vi "HT3_Create.vi"(4 "Image Header in":T3, 5 "Save pt3":bool=TRUE, 6 "Measurement Type":T2(ring)=enum."Point Measurement", 7 "overwrite existing":bool, 8 "error in":errorcluster, 9 "Comment":string, 10 "ht3 Header in":T4={"Comment"="", "Binning"=0, "Offset"=0, "AcquisitionTime (ms)"=0, "HardwareSerial"=0, "SyncDivider"=0, "Resolution (ps)"=0.0, "InpRate0"=0, "InpRate1"=0, "CFD Settings"={"Sync Level"=150, "Sync ZeroX"=10, "Sync Offset"=-1000, "Chan Settings"=[{"CHx Level"=50, "CHx ZeroX"=10, "CHx Offset"=0}, {"CHx Level"=50, "CHx ZeroX"=10, "CHx Offset"=0}, {"CHx Level"=50, "CHx ZeroX"=10, "CHx Offset"=0}, {"CHx Level"=50, "CHx ZeroX"=10, "CHx Offset"=0}]}, "ModuleInfo"=[], "BaseResolution (ps)"=0.0, "RefClockSource"=0, "ChanInfo"=[], "SyncRate"=0, "InputsEnabled"=0}, 11 "File Path":path) -> (0 "error out":errorcluster, 2 "FileHeaderPos":T1, 3 "refnum out":refnum<file>)   [LabVIEW 2013]
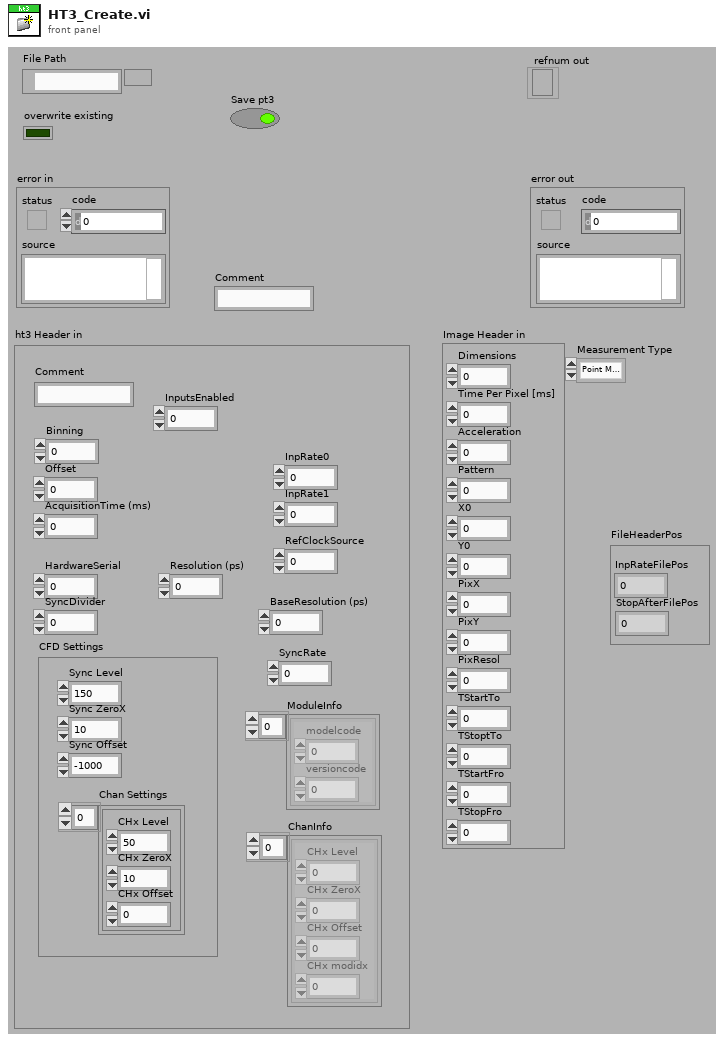
[diagram p1: front panel]
types:
  T1 = cluster{"InpRateFilePos":i64, "StopAfterFilePos":i64}
  T2 = enum16{"not a pt3 File", "Image File", "Point Measurement", "Auto Point", "Line Scan"}
  T3 = cluster{"Dimensions":i32, "Time Per Pixel [ms]":dbl, "Acceleration":i32, "Pattern":i32, "X0":sgl, "Y0":sgl, "PixX":i32, "PixY":i32, "PixResol":sgl, "TStartTo":sgl, "TStoptTo":sgl, "TStartFro":sgl, "TStopFro":sgl}
  T4 = cluster{"Comment":string, "Binning":i32, "Offset":i32, "AcquisitionTime (ms)":i32, "HardwareSerial":i32, "SyncDivider":i32, "Resolution (ps)":dbl, "InpRate0":i32, "InpRate1":i32, "CFD Settings":cluster{"Sync Level":i32, "Sync ZeroX":i32, "Sync Offset":i32, "Chan Settings":cluster{"CHx Level":i32, "CHx ZeroX":i32, "CHx Offset":i32}[]}, "ModuleInfo":cluster{"modelcode":i32, "versioncode":i32}[], "BaseResolution (ps)":dbl, "RefClockSource":i32, "ChanInfo":cluster{"CHx Level":i32, "CHx ZeroX":i32, "CHx Offset":i32, "CHx modidx":i32}[], "SyncRate":i32, "InputsEnabled":i64}
  T5 = enum16{"big-endian, network order", "native, host order", "little-endian"}
  T6 = enum16{"open", "replace", "create", "open or create", "replace or create", "replace or create with confirmation"}
  T7 = cluster{"NumberOfCurves":i32, "Bits per Record":i32, "ActiveCurve":i32, "MeasurementMode (3 = T3)":i32, "f":i32, "Binning":i32, "Resolution (ps)":dbl, "Offset":i32, "AcquisitionTime (ms)":i32, "StopAt":u32, "StopOnOvfl":i32, "Restart":i32, "DisplayLinLog":i32, "DisplayTimeAxisFrom":i32, "DisplayTimeAxisTo":i32, "DisplayCountAxisFrom":i32, "DisplayCountAxisTo":i32}
  T8 = cluster{"Sync Level":i32, "Sync ZeroX":i32, "Sync Offset":i32, "Chan Settings":cluster{"CHx Level":i32, "CHx ZeroX":i32, "CHx Offset":i32}[]}
  T9 = cluster{"CHx Level":i32, "CHx ZeroX":i32, "CHx Offset":i32, "CHx modidx":i32}[]
  T10 = cluster{"BaseResolution (ps)":dbl, "InputsEnabled":i64, i32, "RefClockSource":i32, "ExtDevices":i32, "MarkerSettings":i32, "SyncDivider":i32, "Sync Level":i32, "Sync ZeroX":i32, "Sync Offset":i32}
  T11 = cluster{"SyncRate":i32, "StopAfter":i32, "StopReason":i32, "f":i32, "NumRecords":i64}
  T12 = cluster{"offset (in bytes)":i64, "offset (in bytes)":i64}
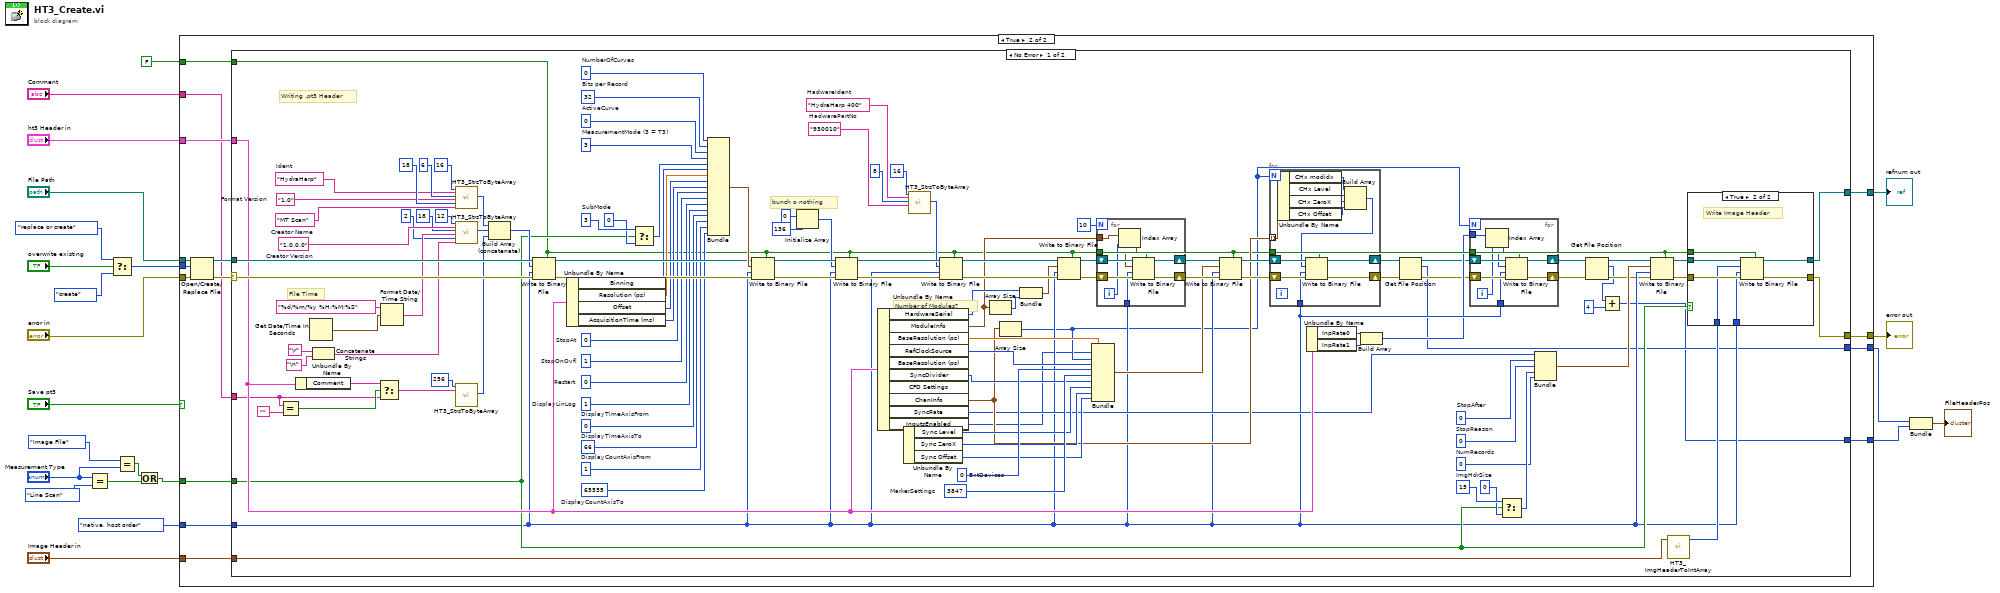
[diagram p0: block diagram]
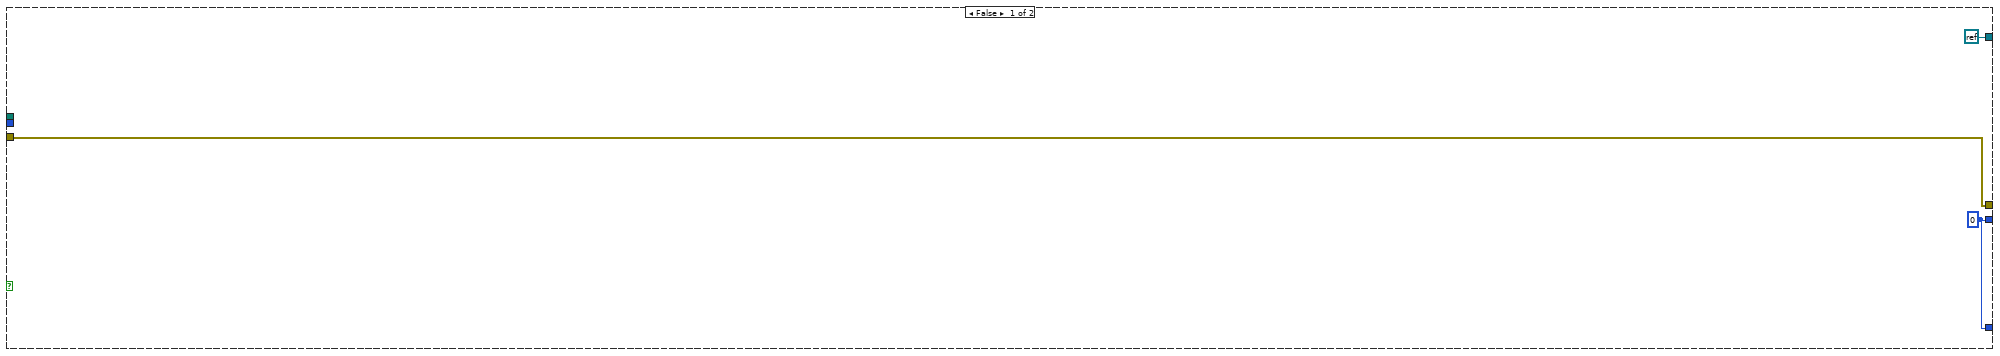
[diagram p2: hidden frame]
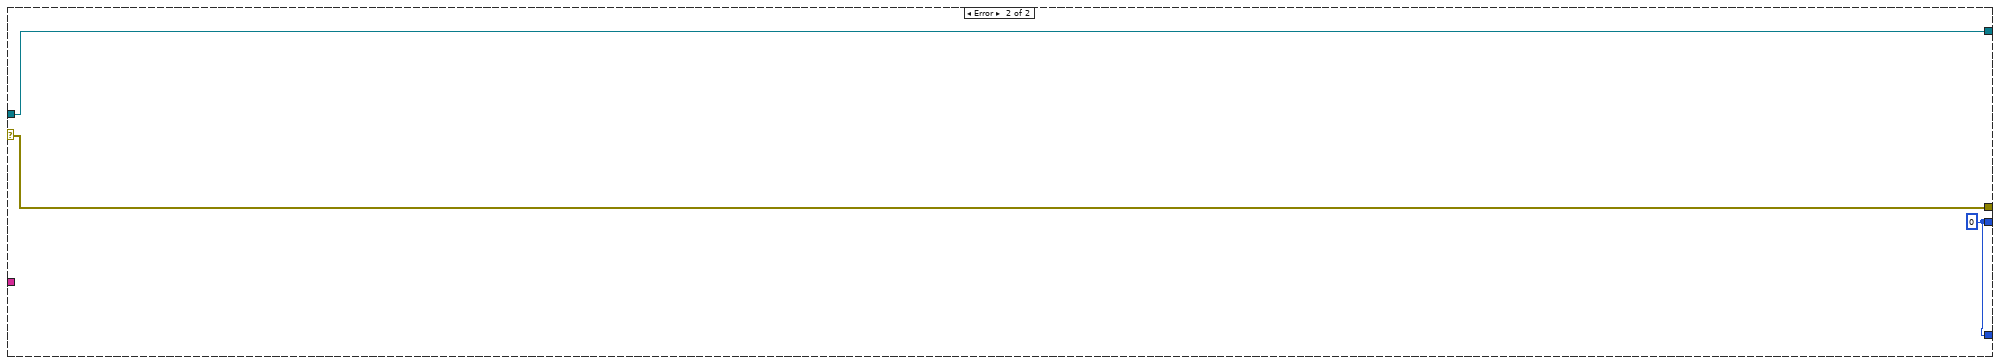
[diagram p4: hidden frame]
diagram:
  n1 = Equal?(x="Measurement Type", y=T2."Line Scan") -> (x = y?=w3:bool)
  n2 = Select(t=T6."replace or create" ("operation (0:open)"), s="overwrite existing", f=T6."create" ("operation (0:open)")) -> (s? t:f=w19:T6)
  n3 = Equal?(x=T2."Image File" ("y"), y="Measurement Type") -> (x = y?=w2:bool)
  n4 = Or(x=w2, y=w3) -> (x .or. y?=w1:bool)
  n5 = case shown="True" "Save pt3" {
    tunnel: "File Path" -> [_ w41]
    tunnel: w19 -> [_ w40]
    tunnel: "error in" -> [w26 w39]
    tunnel: [w26 w37] -> w17
    tunnel: [refnum<k0> refnum w35] -> w16
    tunnel: "ht3 Header in" -> [_ w34]
    tunnel: T5."native, host order" ("byte order (0:big-endian, network order)") -> [_ w33]
    tunnel: FALSE ("prepend array or string size? (T)") -> [_ w32]
    tunnel: "Comment" -> [_ w31]
    tunnel: w1 -> [_ w30]
    tunnel: "Image Header in" -> [_ w29]
    tunnel: [w24 w28] -> w9
    tunnel: [w24 w27] -> w8
    frame False {
      w24 = i64 0 ("offset (in bytes)")
    }
    frame True {
      n6 = Open/Create/Replace File(file path (use dialog)=w41, error in=w39, operation (0:open)=w40) -> (refnum out=w36:refnum<file>, error out=w38:errorcluster)  [unwired: 4 out]
      n7 = case shown="No Error" w38 {
        selector: w38 -> [w162 w204]
        tunnel: [w91 w204] -> w37
        tunnel: w36 -> [w161 w203]
        tunnel: [w89 w203] -> w35
        tunnel: w34 -> [w107 _]
        tunnel: w33 -> [w58 _]
        tunnel: w32 -> [w59 _]
        tunnel: w31 -> [w100 _]
        tunnel: w30 -> [w93 _]
        tunnel: w29 -> [w94 _]
        tunnel: [w44 w202] -> w28
        tunnel: [w43 w202] -> w27
        frame No Error {
          w74 = 3847  # MarkerSettings
          w75 = 0  # ExtDevices
          w96 = 15  # ImgHdrSize
          w60 = i64 0  # NumRecords
          w105 = 0  # StopReason
          w106 = 0  # StopAfter
          w113 = "930010"  # HadwarePartNo
          w115 = "HydraHarp 400"  # HadwareIdent
          w124 = 65535  # DisplayCountAxisTo
          w125 = 1  # DisplayCountAxisFrom
          w126 = 66  # DisplayTimeAxisTo
          w127 = 0  # DisplayTimeAxisFrom
          w128 = 1  # DisplayLinLog
          w129 = 0  # Restart
          w130 = 1  # StopOnOvfl
          w131 = u32 0  # StopAt
          w98 = 3  # SubMode
          w135 = 3  # MeasurementMode (3 = T3)
          w136 = 0  # ActiveCurve
          w86 = 32  # Bits per Record
          w87 = 0  # NumberOfCurves
          w150 = "1.0.0.0"  # Creator Version
          w151 = "MT Scan"  # Creator Name
          w152 = "1.0"  # Format Version
          w153 = "HydraHarp"  # Ident
          # "Number of Modules?"
          # "bunch o nothing"
          # "File Time"
          # "Writing .pt3 Header"
          n8 = Equal?(x=w100, y="") -> (x = y?=w102:bool)
          n9 = Unbundle By Name(w107) -> ("Comment"=w101:string)
          n10 = Get Date/Time In Seconds() -> (seconds since 1Jan1904=w158:timestamp)
          n11 = Concatenate Strings("\r", "\n") -> (w148:string)
          n12 = Select(t=w101, s=w102, f=w100) -> (s? t:f=w99:string)
          n13 = Format Date/Time String(time format string (%c)="%d/%m/%y %H:%M:%S", seconds (now)=w158) -> (date/time string=w149:string)  [unwired: 1 out]
          n14 = call "HT3_StrsToByteArray.vi"("Length"=16, "String"=w153, "Length 2"=6 ("Length"), "String 2"=w152, "Length 3"=18 ("Length"), "String 3"=w151) -> ("Byte Array"=w144:u8[])  [unwired: 1 in, 12 out]
          n15 = call "HT3_StrsToByteArray.vi"("Length"=12, "String"=w150, "Length 2"=18 ("Length"), "String 2"=w149, "Length 3"=2 ("Length"), "String 3"=w148) -> ("Byte Array"=w143:u8[])  [unwired: 1 in, 12 out]
          n16 = call "HT3_StrsToByteArray.vi"("Length"=256, "String"=w99) -> ("Byte Array"=w141:u8[])  [unwired: 5 in, 12 out]
          n17 = Build Array (concatenate)(w144, w143, w141) -> (w140:u8[])
          n18 = Write to Binary File(file (use dialog)=w161, data=w140, error in=w162, 5:w59, 9:w58) -> (refnum out=w137:refnum<file>, error out=w138:errorcluster)  [unwired: 2 out]
          n19 = Unbundle By Name(w107) -> ("Binning"=w84:i32, "Resolution (ps)"=w134:dbl, "Offset"=w133:i32, "AcquisitionTime (ms)"=w132:i32)
          n20 = Select(t=w98, s=w93, f=0) -> (s? t:f=w85:i32)
          n21 = Bundle("NumberOfCurves"=w87, "Bits per Record"=w86, "ActiveCurve"=w136, "MeasurementMode (3 = T3)"=w135, "f"=w85, "Binning"=w84, "Resolution (ps)"=w134, "Offset"=w133, "AcquisitionTime (ms)"=w132, "StopAt"=w131, "StopOnOvfl"=w130, "Restart"=w129, "DisplayLinLog"=w128, "DisplayTimeAxisFrom"=w127, "DisplayTimeAxisTo"=w126, "DisplayCountAxisFrom"=w125, "DisplayCountAxisTo"=w124) -> (w139:T7)  [unwired: 1 in]
          n22 = Write to Binary File(file (use dialog)=w137, data=w139, error in=w138, 5:w59, 9:w58) -> (refnum out=w122:refnum<file>, error out=w123:errorcluster)  [unwired: 2 out]
          n23 = Initialize Array(u8 0 ("element"), 136 ("dimension size")) -> (w119:u8[])
          n24 = Write to Binary File(file (use dialog)=w122, data=w119, error in=w123, 5:w59, 9:w58) -> (refnum out=w117:refnum<file>, error out=w118:errorcluster)  [unwired: 2 out]
          n25 = Unbundle By Name(w107) -> ("HardwareSerial"=w109:i32, "ModuleInfo"=w78:cluster{"modelcode":i32, "versioncode":i32}[], "BaseResolution (ps)"=w77:dbl, "RefClockSource"=w76:i32, "SyncDivider"=w73:i32, "CFD Settings"=w72:T8, "ChanInfo"=w65:T9, "SyncRate"=w62:i32, "InputsEnabled"=w55:i64)  [unwired: 1 out]
          n26 = Unbundle By Name(w72) -> ("Sync Level"=w71:i32, "Sync ZeroX"=w70:i32, "Sync Offset"=w69:i32)
          n27 = call "HT3_StrsToByteArray.vi"("Length"=16, "String"=w115, "Length 2"=8, "String 2"=w113) -> ("Byte Array"=w116:u8[])  [unwired: 3 in, 12 out]
          n28 = Write to Binary File(file (use dialog)=w117, data=w116, error in=w118, 5:w59, 9:w58) -> (refnum out=w110:refnum<file>, error out=w111:errorcluster)  [unwired: 2 out]
          n29 = Array Size(array=w78) -> (size(s)=w79:i32)
          n30 = Array Size(array=w65) -> (size(s)=w56:i32)
          n31 = Bundle("HardwareSerial"=w109, w79) -> (w108:cluster{"HardwareSerial":i32, i32})  [unwired: 1 out]
          n32 = Write to Binary File(file (use dialog)=w110, data=w108, error in=w111, 5:w59, 9:w58) -> (refnum out=w83:refnum<file>, error out=w82:errorcluster)  [unwired: 2 out]
          n33 = Bundle("BaseResolution (ps)"=w77, "InputsEnabled"=w55, w56, "RefClockSource"=w76, "ExtDevices"=w75, "MarkerSettings"=w74, "SyncDivider"=w73, "Sync Level"=w71, "Sync ZeroX"=w70, "Sync Offset"=w69) -> (w68:T10)  [unwired: 1 in]
          n34 = for {
            N: 10 -> [_]
            tunnel: w59 -> [w188]
            shift-right: [w189] -> w80
            shift-left: w83 -> [w192]
            shift-right: [w190] -> w81
            shift-left: w82 -> [w191]
            tunnel: w78 -> [w186]
            tunnel: w58 -> [w187]
            i -> [w185]
            n35 = Index Array(array=w186, index=w185) -> (element=w184:cluster{"modelcode":i32, "versioncode":i32})
            n36 = Write to Binary File(file (use dialog)=w192, data=w184, error in=w191, 5:w188, 9:w187) -> (refnum out=w189:refnum<file>, error out=w190:errorcluster)  [unwired: 2 out]
          }
          n37 = Write to Binary File(file (use dialog)=w80, data=w68, error in=w81, 5:w59, 9:w58) -> (refnum out=w67:refnum<file>, error out=w66:errorcluster)  [unwired: 2 out]
          n38 = for {
            N: w56 -> [_]
            tunnel: w59 -> [w179]
            shift-right: [w180] -> w54
            shift-left: w67 -> [w183]
            shift-right: [w181] -> w53
            shift-left: w66 -> [w182]
            tunnel: w65 -> [w177] mode=indexing
            tunnel: w58 -> [w178]
            n39 = Unbundle By Name(w177) -> ("CHx modidx"=w176:i32, "CHx Level"=w175:i32, "CHx ZeroX"=w174:i32, "CHx Offset"=w173:i32)
            n40 = Build Array(w176, w175, w174, w173) -> (w172:i32[])
            n41 = Write to Binary File(file (use dialog)=w183, data=w172, error in=w182, 5:w179, 9:w178) -> (refnum out=w180:refnum<file>, error out=w181:errorcluster)  [unwired: 2 out]
          }
          n42 = Unbundle By Name(w107) -> ("InpRate0"=w64:i32, "InpRate1"=w63:i32)
          n43 = Build Array(w64, w63) -> (w57:i32[])
          n44 = Get File Position(4:w53, 7:w54) -> (0:w52:errorcluster, 2:w44:i64, 3:w51:refnum<file>)
          n45 = for {
            N: w56 -> [_]
            tunnel: w59 -> [w167]
            shift-right: [w168] -> w49
            shift-left: w51 -> [w171]
            shift-right: [w169] -> w50
            shift-left: w52 -> [w170]
            tunnel: w57 -> [w165]
            tunnel: w58 -> [w166]
            i -> [w164]
            n46 = Index Array(array=w165, index=w164) -> (element=w163:i32)
            n47 = Write to Binary File(file (use dialog)=w171, data=w163, error in=w170, 5:w167, 9:w166) -> (refnum out=w168:refnum<file>, error out=w169:errorcluster)  [unwired: 2 out]
          }
          n48 = Select(t=w96, s=w93, f=0) -> (s? t:f=w61:i32)
          n49 = Bundle("SyncRate"=w62, "StopAfter"=w106, "StopReason"=w105, "f"=w61, "NumRecords"=w60) -> (w104:T11)  [unwired: 1 in]
          n50 = Get File Position(4:w50, 7:w49) -> (0:w47:errorcluster, 2:w46:i64, 3:w48:refnum<file>)
          n51 = Add(x=w46, y=i64 4) -> (x+y=w43:i64)
          n52 = Write to Binary File(file (use dialog)=w48, data=w104, error in=w47, 5:w59, 9:w58) -> (refnum out=w90:refnum<file>, error out=w92:errorcluster)  [unwired: 2 out]
          n53 = call "HT3_ImgHeaderToIntArray.vi"("Image Header"=w94) -> ("Array"=w88:i32[])  [unwired: 10 out]
          n54 = case shown="True" w93 {
            tunnel: w92 -> [w193 w201]
            tunnel: [w193 w200] -> w91
            tunnel: w90 -> [w194 w199]
            tunnel: [w194 w198] -> w89
            tunnel: w59 -> [_ w197]
            tunnel: w88 -> [_ w196]
            tunnel: w58 -> [_ w195]
            frame False {
            }
            frame True {
              # "Write Image Header"
              n55 = Write to Binary File(file (use dialog)=w199, data=w196, error in=w201, 5:w197, 9:w195) -> (refnum out=w198:refnum<file>, error out=w200:errorcluster)  [unwired: 2 out]
            }
          }
        }
        frame Error {
          w202 = i64 0 ("offset (in bytes)")
        }
      }
    }
  }
  "refnum out" <- w16
  "error out" <- w17
  n56 = Bundle("offset (in bytes)"=w9, "offset (in bytes)"=w8) -> (→"FileHeaderPos":T12)  [unwired: 1 in]
